vi "subLogger.vi"(1 "Clear Flag":bool, 2 "Description":string, 3 "User Level":i32, 4 "Value":string, 5 "Location":string, 6 "Level":string) -> (0 "To Screen":string)   [LabVIEW 2017]
panel:
  in  "User Level String":string
  out "Old Location":string
  out "Old Value":string
  out "path":path
  out "error out":errorcluster
  in  "error in (no error)":errorcluster
  # "This VI gathers received string information\nand concatenates them into a standardised\nlogging format to then be printed to logs. It also\nchecks against the same condition being sent\nfrom the same log location twice to prevent\nconstant logging for the same event."
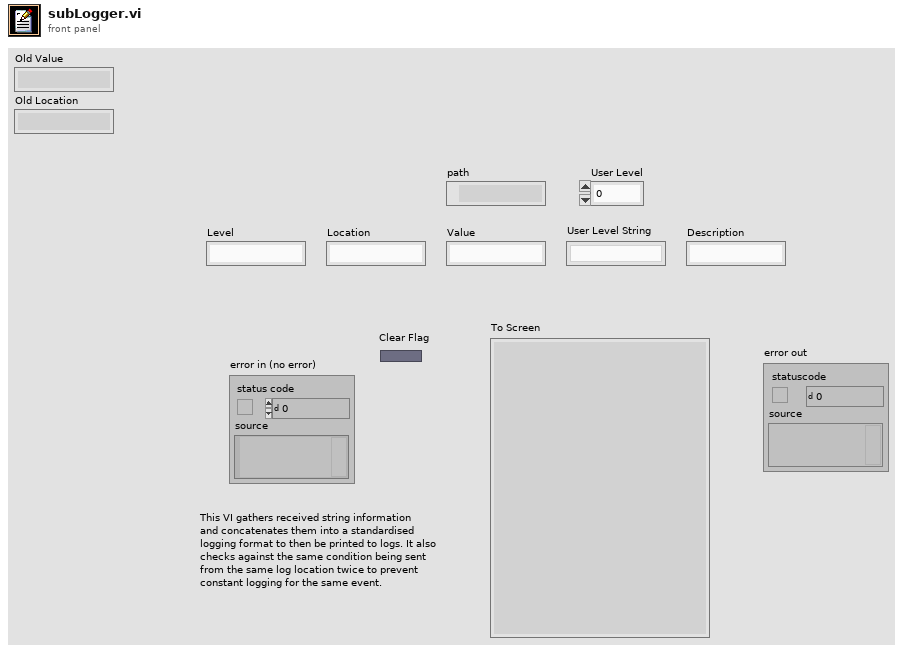
[diagram p1: front panel]
types:
  T1 = enum16{"open", "replace", "create", "open or create", "replace or create", "replace or create with confirmation"}
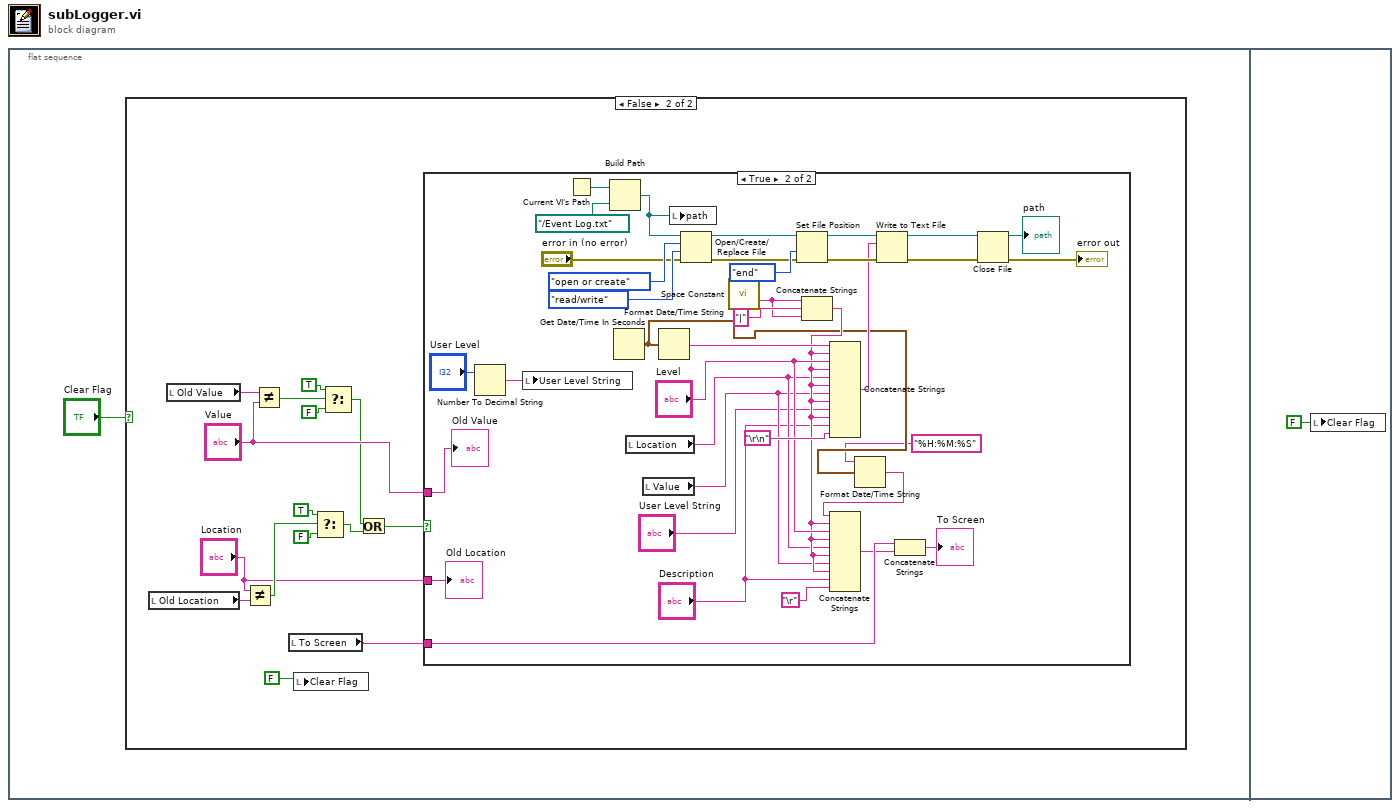
[diagram p0: block diagram]
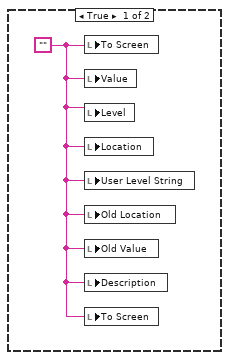
[diagram p2: hidden frame]
diagram:
  n1 = flat-sequence {
    frame #0 {
      n2 = case shown="False" "Clear Flag" {
        frame True {
          w2 = ""
          n3 = local write "To Screen"(w2) -> ()
          n4 = local write "Value"(w2) -> ()
          n5 = local write "Level"(w2) -> ()
          n6 = local write "Location"(w2) -> ()
          n7 = local write "User Level String"(w2) -> ()
          n8 = local write "Old Location"(w2) -> ()
          n9 = local write "Old Value"(w2) -> ()
          n10 = local write "Description"(w2) -> ()
          n11 = local write "To Screen"(w2) -> ()
        }
        frame False {
          n12 = local read "Old Location"() -> (w17:string)
          n13 = local read "Old Value"() -> (w9:string)
          n14 = Not Equal?(x="Location", y=w17) -> (x != y?=w16:bool)
          n15 = Not Equal?(x=w9, y="Value") -> (x != y?=w6:bool)
          n16 = local read "To Screen"() -> (w4:string)
          n17 = local write "Clear Flag"(FALSE) -> ()
          n18 = Select(t=TRUE, s=w16, f=FALSE) -> (s? t:f=w10:bool)
          n19 = Select(t=TRUE, s=w6, f=FALSE) -> (s? t:f=w5:bool)
          n20 = Or(x=w5, y=w10) -> (x .or. y?=w12:bool)
          n21 = case shown="True" w12 {
            tunnel: "Value" -> [_ w37]
            tunnel: "Location" -> [_ w35]
            tunnel: w4 -> [_ w24]
            frame False {
            }
            frame True {
              n22 = Number To Decimal String(number="User Level") -> (decimal integer string=w21:string)  [unwired: 1 in]
              n23 = local write "User Level String"(w21) -> ()
              n24 = Current VI's Path() -> (path=w54:path)
              n25 = Build Path(base path=w54, name or relative path=path "../Event Log.txt") -> (appended path=w47:path)
              n26 = Get Date/Time In Seconds() -> (seconds since 1Jan1904=w20:timestamp)
              n27 = local read "Location"() -> (w29:string)
              n28 = local read "Value"() -> (w28:string)
              n29 = Format Date/Time String(seconds (now)=w20) -> (date/time string=w32:string)  [unwired: 2 in]
              n30 = local write "path"(w47) -> ()
              n31 = Open/Create/Replace File(file path (use dialog)=w47, error in="error in (no error)", operation (0:open)=T1."open or create", access (0:read/write)=enum16{"read/write", "read-only", "write-only"}."read/write") -> (refnum out=w43:refnum<file>, error out=w40:errorcluster)  [unwired: 2 in, 1 out]
              n32 = call <vilib>:"Space Constant.vi"() -> ("String"=w34:string)
              n33 = Set File Position(refnum=w43, from (0:start)=enum16{"start", "end", "current"}."end", error in=w40) -> (refnum out=w42:refnum<file>, error out=w39:errorcluster)  [unwired: 1 in]
              n34 = Concatenate Strings(w34, "|", w34) -> (w30:string)
              n35 = Concatenate Strings(w32, w30, "Level", w30, w29, w30, w28, w30, "User Level String", w30, "Description", "\r\n") -> (w33:string)
              n36 = Format Date/Time String(time format string (%c)="%H:%M:%S", seconds (now)=w20) -> (date/time string=w19:string)  [unwired: 1 in]
              n37 = Concatenate Strings(w19, w30, "Level", w30, w29, w30, w28, w30, "Description", "\r") -> (w23:string)
              n38 = Write to Text File(file (use dialog)=w42, text=w33, error in=w39) -> (refnum out=w46:refnum<file>, error out=w45:errorcluster)  [unwired: 1 in, 1 out]
              n39 = Concatenate Strings(w24, w23) -> (→"To Screen":string)
              n40 = Close File(refnum=w46, error in=w45) -> (path=→"path":path, error out=→"error out":errorcluster)
              "Old Value" <- w37
              "Old Location" <- w35
            }
          }
        }
      }
    }
    frame #1 {
      n41 = local write "Clear Flag"(FALSE) -> ()
    }
  }
